vi "filetest.vi"() -> ()   [LabVIEW 2019]
uses:
  <vilib>/userDefined/High Color/IMAQdx.ctl
  <vilib>/vision/driver/NI_Vision_Acquisition_Software.lvlib
panel:
  out "Image":T1(plugin-control)
  in  "stop":bool
  out "Image 2":T1(plugin-control)
  out "String (OCR/OCV 1)":string
  in  "File Path (OCR/OCV 1)":path=path "D:/3下課程/總結式課程/影像/OCR/train1.abc"
  out "number":i32
  out "100":dbl
  out "10":dbl
  out "1":dbl
  out "Boolean":bool
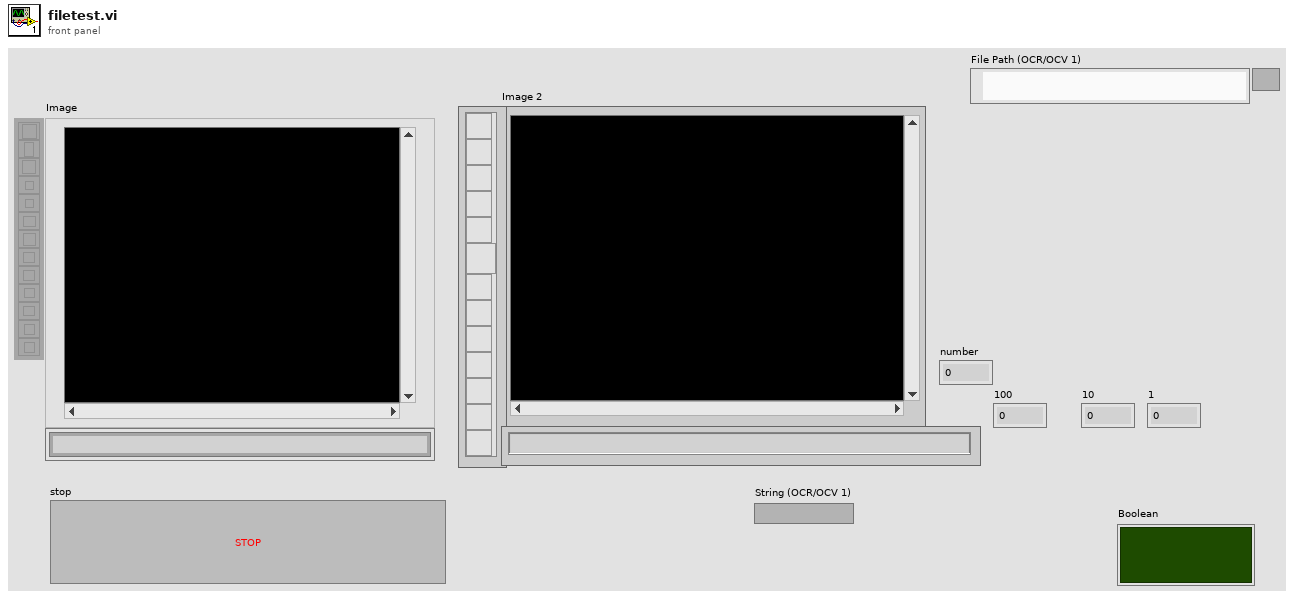
[diagram p1: front panel]
types:
  T1 = typedef "IMAQ Image.ctl" = refnum<image>
  T2 = typedef "IMAQdx.ctl" = refnum<k21>
  T3 = typedef "IMAQ Rectangle" = cluster{"Left":i32, "Top":i32, "Right":i32, "Bottom":i32, "Rotation":dbl}
  T4 = typedef "ROI Descriptor" = cluster{"Global Rectangle":i32[], "Contours":cluster{"ID":enum32{"External", "Internal"}, "Type":u32, "Coordinates":i32[]}[]}
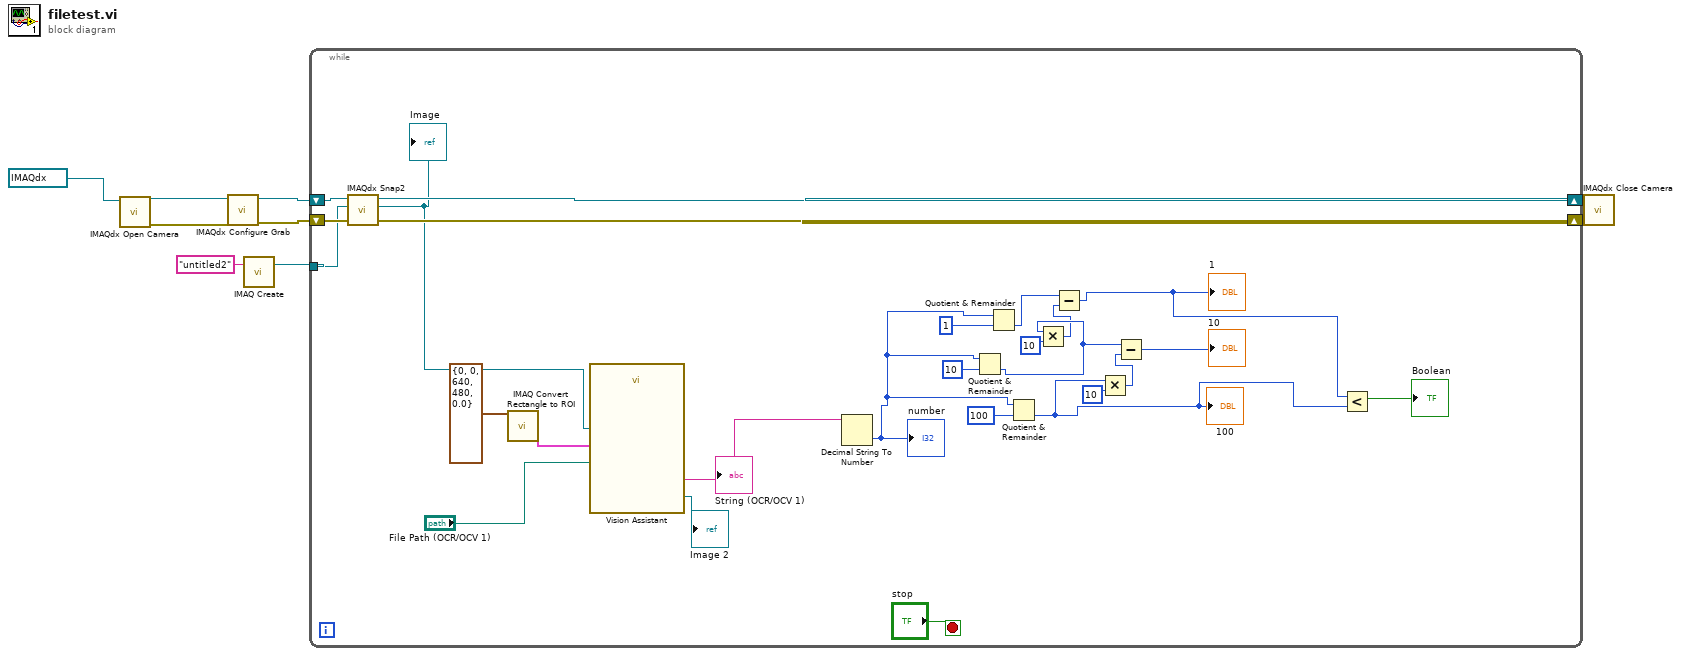
[diagram p0: block diagram]
diagram:
  n1 = call <vilib>:"IMAQdx Open Camera.vi"("Session In"=T2 "cam0") -> ("error out"=w5:errorcluster, "Session Out"=w8:T2)  [unwired: 9 in]
  n2 = call <vilib>:"IMAQdx Configure Grab.vi"("error in"=w5, "Session In"=w8) -> ("error out"=w4:errorcluster, "Session Out"=w7:T2)  [unwired: 8 in]
  n3 = call "IMAQ Create"("Image Name"="untitled2") -> ("New Image"=w1:T1)  [unwired: 4 in, 1 out]
  n4 = while {
    tunnel: w1 -> [w29]
    shift-right: [w34] -> w6
    shift-left: w7 -> [w35]
    shift-right: [w32] -> w3
    shift-left: w4 -> [w33]
    stop <- "stop" stop-if-true
    n5 = call <vilib>:"IMAQdx Snap2.vi"("error in"=w33, "Image In"=w29, "Session In"=w35) -> ("error out"=w32:errorcluster, "Image Out"=w26:T1, "Session Out"=w34:T2)  [unwired: 6 in]
    "Image" <- w26
    n6 = call "IMAQ Convert Rectangle to ROI"("Rectangle"=T3 {"Left"=0, "Top"=0, "Right"=640, "Bottom"=480, "Rotation"=0.0}) -> ("ROI Descriptor"=w27:T4)  [unwired: 8 in, 1 out]
    n7 = call "Vision Assistant"("Image In"=w26, "ROI Descriptor (OCR/OCV 1)"=w27, "File Path (OCR/OCV 1)"="File Path (OCR/OCV 1)") -> ("Image Out"=→"Image 2":T1, "String (OCR/OCV 1)"=w14:string)  [unwired: 22 in, 1 out]
    "String (OCR/OCV 1)" <- w14
    n8 = Decimal String To Number(string=w14) -> (number=w24:i32)  [unwired: 2 in, 1 out]
    "number" <- w24
    n9 = Quotient & Remainder(x=w24, y=10) -> (floor(x/y)=w25:i32)  [unwired: 1 out]
    n10 = Quotient & Remainder(x=w24, y=1) -> (floor(x/y)=w20:i32)  [unwired: 1 out]
    n11 = Quotient & Remainder(x=w24, y=100) -> (floor(x/y)=w12:i32)  [unwired: 1 out]
    "100" <- w12
    n12 = Multiply(x=w25, y=10) -> (x*y=w21:i32)
    n13 = Subtract(x=w20, y=w21) -> (x-y=w13:i32)
    "1" <- w13
    n14 = Multiply(x=w12, y=10) -> (x*y=w22:i32)
    n15 = Subtract(x=w25, y=w22) -> (x-y=→"10":i32)
    n16 = Less?(x=w13, y=w12) -> (x < y?=→"Boolean":bool)
  }
  n17 = call <vilib>:"IMAQdx Close Camera.vi"("error in"=w3, "Session In"=w6) -> ()  [unwired: 9 in, 1 out]
